vi "Build LocalAppData Path.vi"(8 "error in (no error)":errorcluster, 10 "Operating System":string, 11 "Relative path":path) -> (0 "error out":errorcluster, 3 "Full Path":path)   [LabVIEW 2020, in "RxnRover.lvlib" / "File IO.lvlib"]
doc: "Builds a file path with relative path and Local App Data Base Path\nAn Operating system must be specified\nSupports: Windows 2000 - Windows 11, Linux, Mac OS\n\nCreated 5/20/2025 - Labview 2020\nRxnRover"
uses:
  File IO.lvlib
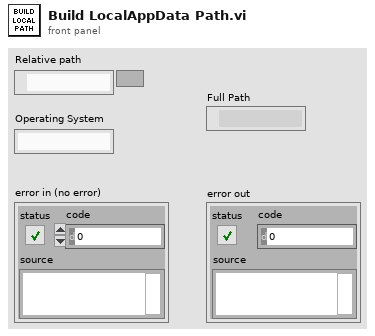
[diagram p1: front panel]
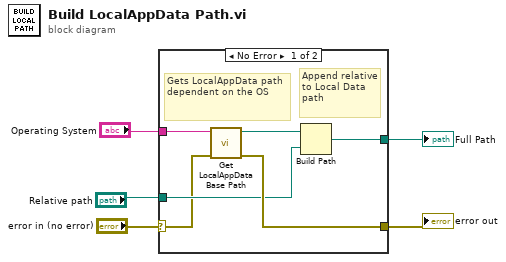
[diagram p0: block diagram]
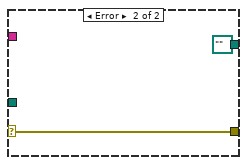
[diagram p2: hidden frame]
diagram:
  n1 = case shown="No Error" "error in (no error)" {
    selector: "error in (no error)" -> [w6 w13]
    tunnel: [w11 w13] -> w5
    tunnel: [w10 path "" ("appended path")] -> w4
    tunnel: "Relative path" -> [w8 _]
    tunnel: "Operating System" -> [w7 _]
    frame No Error {
      # "Gets LocalAppData path dependent on the OS"
      # "Append relative to Local Data path"
      n2 = call "Get LocalAppData Base Path.vi"("error in (no error)"=w6, "Operating System"=w7) -> ("error out"=w11:errorcluster, "Path"=w9:path)  [unwired: 8 in]
      n3 = Build Path(base path=w9, name or relative path=w8) -> (appended path=w10:path)
    }
    frame Error {
    }
  }
  "error out" <- w5
  "Full Path" <- w4
